vi "Load Joint Velocity.vi"(7 "Units (Encoder Counts)":T3=enum."Encoder Counts", 8 "error in (no error)":errorcluster, 9 "Velocity":dbl, 10 "Axis":T4=1 items=["Axis 1"=1, "Axis 2"=2, "Axis 3"=3, "Axis 4"=4, "Axis 5"=5, "Axis 6"=6, "Axis 7"=7, "Axis 8"=8], 11 "Board ID":T5=1 min=1 max=32 step=1) -> (0 "error out":errorcluster, 2 "Resource Output":T1=1 items=["Axis Control"=0, "Axis 1"=1, "Axis 2"=2, "Axis 3"=3, "Axis 4"=4, "Axis 5"=5, "Axis 6"=6, "Axis 7"=7, "Axis 8"=8, "Vector Space Control"=16, "Vector Space 1"=17, "Vector Space 2"=18, "Vector Space 3"=19, "Vector Space 4"=20, "Encoder Control"=32, "Encoder 1"=33, "Encoder 2"=34, "Encoder 3"=35, "Encoder 4"=36, "Encoder 5"=37, "Encoder 6"=38, "Encoder 7"=39, "Encoder 8"=40, "DAC Channel 1"=49, "DAC Channel 2"=50, "DAC Channel 3"=51, "DAC Channel 4"=52, "DAC Channel 5"=53, "DAC Channel 6"=54, "DAC Channel 7"=55, "DAC Channel 8"=56, "Stepper Output 1"=65, "Stepper Output 2"=66, "Stepper Output 3"=67, "Stepper Output 4"=68, "Stepper Output 5"=69, "Stepper Output 6"=70, "Stepper Output 7"=71, "Stepper Output 8"=72, "ADC Channel 1"=81, "ADC Channel 2"=82, "ADC Channel 3"=83, "ADC Channel 4"=84, "ADC Channel 5"=85, "ADC Channel 6"=86, "ADC Channel 7"=87, "ADC Channel 8"=88], 3 "Bd ID Out":T2)   [LabVIEW 2010]
doc: "Written for the PUMA 560. Loads in the encoder velocity corresponding to the passed in joint velocity for the given axis.\n\nInput units can be specified as either degrees/s (default) or radians/s.\n\nNotes:\n\" Encoder velocity is computed using the formula: edot = thetadot*epr*N/(2*pi)\nWhere thetadot is the joint velocity, N is the gear ratio for the given axis (referenced from [X]), 2*pi is 360 in the case of degrees units, edot is the computed encoder velocity, and epr is the encoder counts per revolution of the axis.\n\" Computed encoder velocity is loaded into controller board with the FlexMotion \"Load Velocity.flx\""
uses:
  <vilib>/Motion/FlexMotion/CustomControls/CustomControls.llb/Axis To Read.flx
  Typedefs/Units_Enum.ctl
  <vilib>/Motion/FlexMotion/CustomControls/CustomControls.llb/Resource Out (Enum).flx
  Globals/AxisSpace.vi
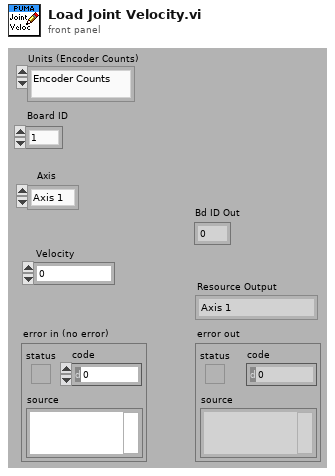
[diagram p1: front panel]
types:
  T1 = typedef "Resource Out (Enum).flx" = u16
  T2 = typedef "Bd Id Out" = u8
  T3 = typedef "Units_Enum.ctl" = enum16{"Radians", "Encoder Counts", "Revolutions", "Degrees"}
  T4 = typedef "Axis To Read.flx" = u16
  T5 = typedef "Board Id" = u8
  T6 = typedef "AxisSpaceCfg_ArrayofAxisCfg.ctl" = T7[]
  T7 = typedef "AxisCfg_cluster.ctl" = cluster{"Axis":T4, "Counts/Rev":dbl, "Gear Ratio":dbl, "Home Position":dbl}
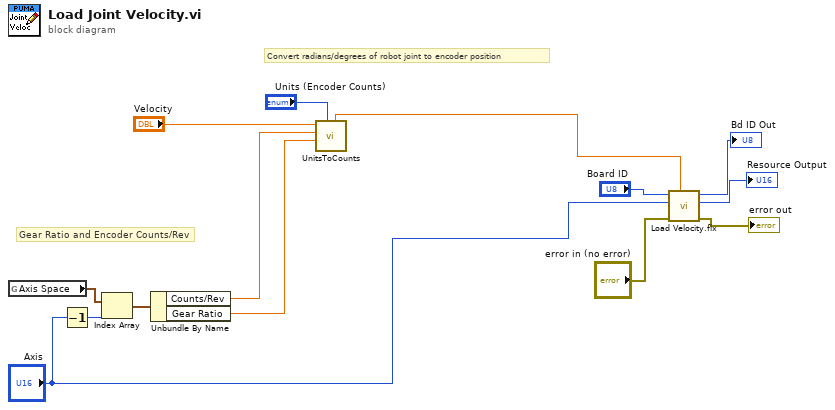
[diagram p0: block diagram]
diagram:
  # "Convert radians/degrees of robot joint to encoder position"
  # "Gear Ratio and Encoder Counts/Rev"
  n1 = global read "AxisSpace.vi" "Axis Space"() -> (w8:T6)
  n2 = Decrement(x="Axis") -> (x-1=w9:T4)
  n3 = Index Array(array=w8, index=w9) -> (element=w7:T7)
  n4 = Unbundle By Name(w7) -> ("Counts/Rev"=w2:dbl, "Gear Ratio"=w1:dbl)
  n5 = call "UnitsToCounts.vi"("Units (Encoder Counts)"="Units (Encoder Counts)", "Gear Ratio"=w1, "Counts/Rev"=w2, "Value"="Velocity") -> ("Encoder Counts"=w4:dbl)  [unwired: 7 in]
  n6 = call <vilib>:"Load Velocity.flx"("Velocity (10000)"=w4, "error in (no error)"="error in (no error)", "Axis or Vector Space"="Axis", "Board ID"="Board ID") -> ("error out"=→"error out":errorcluster, "Resource Output"=→"Resource Output":T1, "Bd ID Out"=→"Bd ID Out":T2)  [unwired: 3 in]
